vi "PreBuild.vi"(8 "error in (no error)":errorcluster, 11 "Build in":refnum<class "AB_Application.lvclass">) -> (0 "error out":errorcluster, 3 "Build out":refnum<class "AB_Application.lvclass">)   [LabVIEW 2020, in "AB_Application.lvclass"]
uses:
  <vilib>/AppBuilder/AB_Classes/Application/AB_Application.lvclass
  e:/builds/penguin/labview/branches/2020/dev/dist/vi.lib/AppBuilder/AB_Classes/TargetFile/AB_Targetfile.lvclass
  e:/builds/penguin/labview/branches/2020/dev/dist/vi.lib/AppBuilder/AB_Classes/Build/AB_Build.lvclass
  <vilib>/AppBuilder/AB_Classes/Application/AB_Application.lvclass/AB_Application.ctl
  <vilib>/AppBuilder/AB_Classes/Application/AB_Web_Service_Overrides.ctl
  <vilib>/AppBuilder/AB_Classes/Build/Misc_Data_Keys.vi
  <vilib>/AppBuilder/AB_Classes/Build/AB_Build.lvclass
  <vilib>/AppBuilder/AB_Classes/TargetFile/AB_Targetfile.lvclass
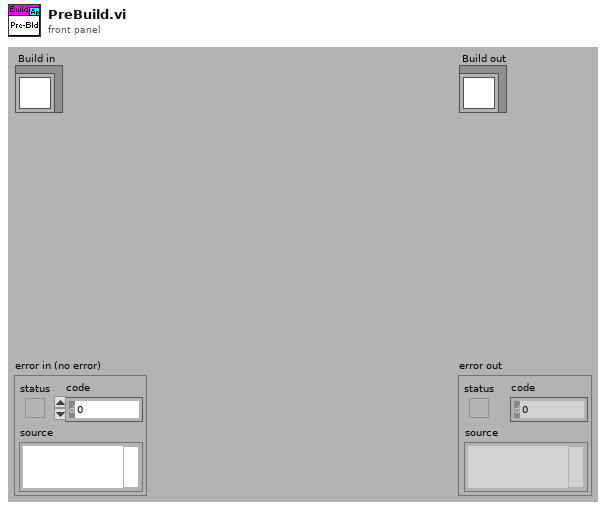
[diagram p1: front panel]
types:
  T1 = typedef "AB_Embedded_Server_Configuration.ctl" = cluster{"HTTP enabled?":bool, "HTTP port":i32, "HTTPS enabled?":bool, "HTTPS port":i32, "SSL certificate file":path}
  T2 = enum32{"NI Web Server", "Application Web Server"}
  T3 = typedef "AB_Web_Service_Overrides.ctl" = cluster{"has overrides?":bool, "debugging?":bool, "modify library?":bool}
  T4 = typedef "AB_Targetfile.ctl" = cluster{"targetfileName":string, "targetfileGUID":string, "enableDebugging":bool, "versionInfo":cluster{"productName":string, "legalCopyright":string, "companyName":string, "internalName":string, "fileDescription":string}, "eng_consolidatedTypeInfo":string, "fastFileFormat":bool, "eng_LEIFBuildData":u32, "versionIndependent":bool}
  T5 = typedef "AB_Build.ctl" = cluster{"buildSpecName":string, "buildSpecDescription":string, "destinations":refnum<class "AB_Destination.lvclass">[], "exclusionOption":T6, "defaultLanguage":string, "supportedLanguages":string[], "excludedDirectories":path[], "buildContext":refnum<vi>, "buildObject":T7, "preview":bool, "programatic":bool, "progressBarEvents":T8, "userLog_Path":path, "preActionID":string, "preAction_Path":path, "postActionID":string, "postAction_Path":path, "eng_checkForBrokenVIs?":bool, "eng_verboseLinkerErrors?":bool, "localDest_Path":path, "targetDest_Path":path, "removeVIObject":u16, "cache":refnum<class "PreviewCache.lvclass">, "use cache":bool, "previewCache_ID":string, "buildCache_ID":string, "eng_TempLocalDest_Path":path, "eng_collectDependencies?":bool, "versionInfo":cluster{"buildVersion":cluster{"major":u16, "minor":u16, "patch":u16, "build":u16}, "autoIncrement":bool}, "eng_enableVIChecksums":bool}
  T6 = typedef "AB_Exclusion_Option.ctl" = cluster{"typedefs":bool, "polymorphicVIs":bool, "unusedLibraryItems":bool, "modifyLibraryFile":bool, "edit-timeDependencies":bool, "inlineVIs":bool, "dependent PPLs":bool, "dependent DLLs":bool}
  T7 = typedef "ItemRef.ctl" = u64
  T8 = typedef "provcom_ProgressBar_Events.ctl" = cluster{"newJob":refnum<user-event>, "newItem":refnum<user-event>, "errorMsg":T9, "cancel":refnum<user-event>}
  T9 = typedef "mxLvBuildError.ctl" = refnum<user-event>
  T10 = enum32{"invalid OS target", "Mac OS", "Windows 3.1", "Windows 95/NT", "Solaris 1", "Solaris 2", "HP-UX", "PowerMAX", "Linux", "Irix", "Rhapsody", "BeOS", "AIX", "OSF1", "VxWorks", "PharLap", "Carbon", "RTX", "Windows x64", "Linux x64", "Mac OS X x64"}
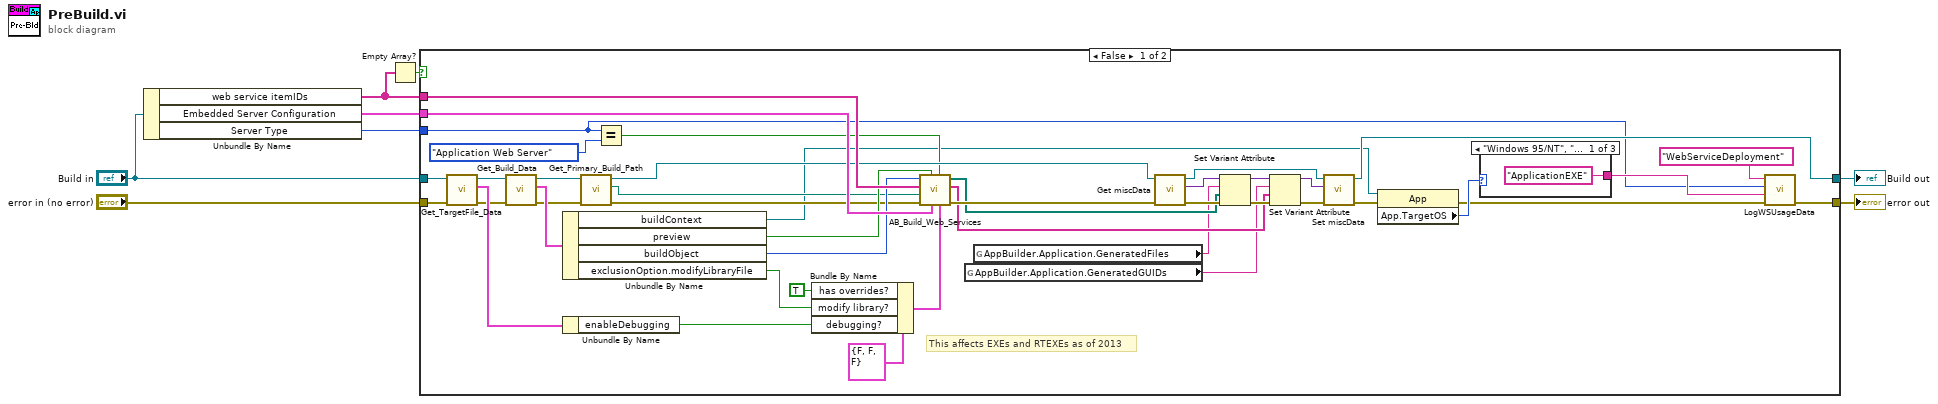
[diagram p0: block diagram]
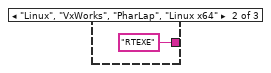
[diagram p2: hidden frame]
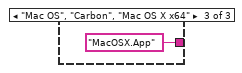
[diagram p3: hidden frame]
diagram:
  n1 = Unbundle By Name("Build in") -> ("web service itemIDs"=w5:string[], "Embedded Server Configuration"=w4:T1, "Server Type"=w1:T2)
  n2 = Empty Array?(array=w5) -> (empty?=w6:bool)
  n3 = case shown="False" w6 {
    tunnel: "error in (no error)" -> [w30 w55]
    tunnel: [w14 w55] -> w8
    tunnel: w5 -> [w42 _]
    tunnel: "Build in" -> [w29 w56]
    tunnel: [w50 w56] -> w7
    tunnel: w4 -> [w39 _]
    tunnel: w1 -> [w9 _]
    frame False {
      # "This affects EXEs and RTEXEs as of 2013"
      n4 = call <vilib>:"Get_TargetFile_Data.vi"("error in (no error)"=w30, "AB_Targetfile in"=w29) -> ("error out"=w25:errorcluster, "data"=w28:T4, "AB_Targetfile out"=w26:refnum<class "AB_Application.lvclass">)  [unwired: 7 in]
      n5 = call <vilib>:"Get_Build_Data.vi"("error in (no error)"=w25, "Class in"=w26) -> ("error out"=w21:errorcluster, "data"=w24:T5, "Class out"=w23:refnum<class "AB_Application.lvclass">)  [unwired: 7 out]
      n6 = Unbundle By Name(w24) -> ("buildContext"=w17:refnum<vi>, "preview"=w33:bool, "buildObject"=w32:T7, "exclusionOption.modifyLibraryFile"=w31:bool)
      n7 = Unbundle By Name(w28) -> ("enableDebugging"=w27:bool)
      n8 = call-dynamic "Get_Primary_Build_Path.vi"("error in (no error)"=w21, "AB_Build in"=w23) -> ("error out"=w20:errorcluster, "Primary build path"=w19:path, "AB_Build out"=w22:refnum<class "AB_Application.lvclass">)  [unwired: 7 in]
      n9 = Equal?(x=w9, y=T2."Application Web Server") -> (x = y?=w18:bool)
      n10 = Bundle By Name(cluster=T3 {"has overrides?"=FALSE, "debugging?"=FALSE, "modify library?"=FALSE} ("Web service overrides"), "has overrides?"=TRUE, "modify library?"=w31, "debugging?"=w27) -> (w35:T3)
      n11 = call <vilib>:"AB_Build_Web_Services.vi"("Web service overrides"=w35, "Generate embedded conf?"=w18, "Embedded Server Configuration"=w39, "Preview?"=w33, "error in (no error)"=w20, "Destination directory"=w19, "web service itemIDs"=w42, "build object"=w32) -> ("error out"=w43:errorcluster, "GeneratedFileGUIDs"=w40:string[], "GeneratedFiles"=w41:path[])  [unwired: 1 in]
      n12 = global read "Misc_Data_Keys.vi" "AppBuilder.Application.GeneratedGUIDs"() -> (w37:string)
      n13 = global read "Misc_Data_Keys.vi" "AppBuilder.Application.GeneratedFiles"() -> (w38:string)
      n14 = call-dynamic "Get miscData.vi"("error in (no error)"=w43, "AB_Build in"=w22) -> ("error out"=w45:errorcluster, "eng_miscData"=w49:variant, "AB_Build out"=w51:refnum<class "AB_Application.lvclass">)  [unwired: 7 in]
      n15 = Set Variant Attribute(Variant=w49, name=w38, value=w41, error in=w45) -> (Variant out=w48:variant, error out=w46:errorcluster)  [unwired: 1 out]
      n16 = Set Variant Attribute(Variant=w48, name=w37, value=w40, error in=w46) -> (Variant out=w47:variant, error out=w44:errorcluster)  [unwired: 1 out]
      n17 = call-dynamic "Set miscData.vi"("error in (no error)"=w44, "eng_miscData"=w47, "AB_Build in"=w51) -> ("error out"=w16:errorcluster, "AB_Build out"=w50:refnum<class "AB_Application.lvclass">)  [unwired: 7 in]
      n18 = property class="App"(reference=w17, error in=w16) -> (error out=w13:errorcluster, "App.TargetOS"=w15:T10)  [unwired: 1 out]
      n19 = case shown="\"Windows 95/NT\", \"Windows x64\", Default" w15 {
        tunnel: ["ApplicationEXE" ("Deploy Method") "RTEXE" ("Deploy Method") "MacOSX.App" ("Deploy Method")] -> w11
        frame "Windows 95/NT", "Windows x64", Default {
        }
        frame "Linux", "VxWorks", "PharLap", "Linux x64" {
        }
        frame "Mac OS", "Carbon", "Mac OS X x64" {
        }
      }
      n20 = call <vilib>:"LogWSUsageData.vi"("Error In"=w13, "Deploy Method"=w11, "Server Type"=w9, "Action"="WebServiceDeployment") -> ("Error Out"=w14:errorcluster)  [unwired: 7 in]
    }
    frame True {
    }
  }
  "error out" <- w8
  "Build out" <- w7
